vi "实验5_4.vi"() -> ()   [LabVIEW 2018]
uses:
  <vilib>/Analysis/NI_AALBase.lvlib
panel:
  in  "Numeric":dbl=20.0
  out "Array":cluster{"Array 2":dbl[], "String":string}[](array[cluster])
  in  "Path":path=path "/Users/fancheyv/Desktop/大三下实验/LabView/file"
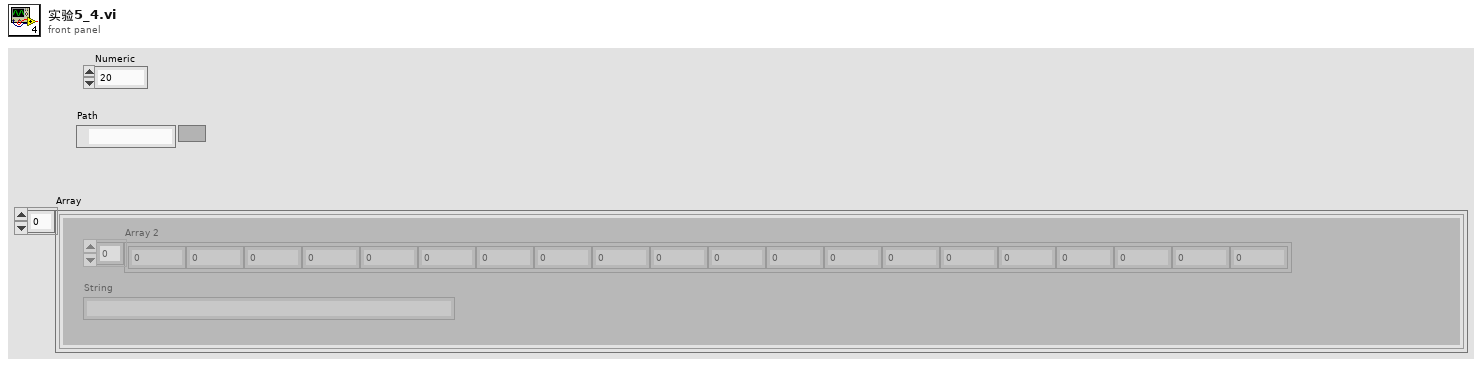
[diagram p1: front panel]
types:
  T1 = enum16{"open", "replace", "create", "open or create", "replace or create", "replace or create with confirmation"}
  T2 = cluster{"periodic random noise":dbl[], "date/time string":string}
  T3 = cluster{"periodic random noise":dbl[], "date/time string":string}[]
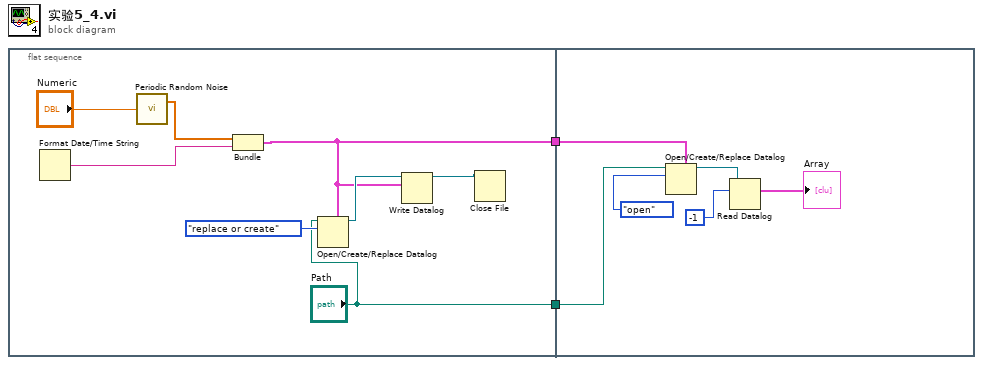
[diagram p0: block diagram]
diagram:
  n1 = flat-sequence {
    tunnel: ["Path"] -> w2
    tunnel: [w4] -> w1
    tunnel: w2 -> [w15]
    tunnel: w1 -> [w12]
    frame #0 {
      n2 = Format Date/Time String() -> (date/time string=w9:string)  [unwired: 3 in]
      n3 = call <vilib>:"Periodic Random Noise.vi"("spectral amplitude"="Numeric") -> ("periodic random noise"=w8:dbl[])  [unwired: 2 in, 1 out]
      n4 = Bundle("periodic random noise"=w8, "date/time string"=w9) -> (w4:T2)  [unwired: 1 in]
      n5 = Open/Create/Replace Datalog(5:w4, 10:T1."replace or create" ("operation (0:open)"), 11:"Path") -> (3:w5:refnum<k1>)  [unwired: 3 in, 2 out]
      n6 = Write Datalog(6:w4, 7:w5) -> (3:w6:refnum<k1>)  [unwired: 1 in, 1 out]
      n7 = Close File(refnum=w6) -> ()  [unwired: 1 in, 2 out]
    }
    frame #1 {
      n8 = Open/Create/Replace Datalog(5:w12, 10:T1."open" ("operation (0:open)"), 11:w15) -> (3:w14:refnum<k1>)  [unwired: 3 in, 2 out]
      n9 = Read Datalog(6:-1, 7:w14) -> (2:→"Array":T3)  [unwired: 1 in, 2 out]
    }
  }
